vi "Stop FGV_redone.vi"(7 "Mode":enum16{"Set", "Get"}(ring), 8 "Error In":errorcluster, 11 "Set Value":bool) -> (0 "Error Out":errorcluster, 3 "Get Value":bool)   [LabVIEW 2018]
doc: "Functional global variable to stop parallel loops."
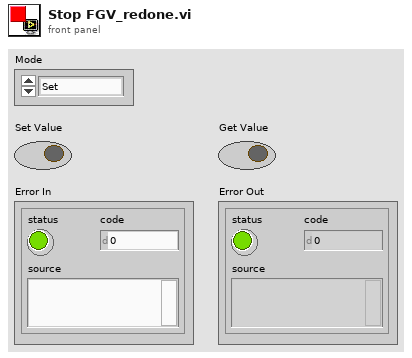
[diagram p1: front panel]
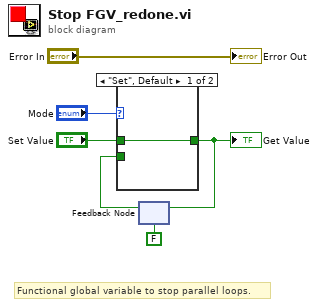
[diagram p0: block diagram]
diagram:
  # "Functional global variable to stop parallel loops."
  n1 = feedback #1(FALSE ("Set Value")) -> (w2:bool)
  n2 = case shown="\"Set\", Default" "Mode" {
    tunnel: "Set Value" -> [w7 _]
    tunnel: [w7 w8] -> w3
    tunnel: w2 -> [_ w8]
    frame "Set", Default {
    }
    frame "Get" {
    }
  }
  "Get Value" <- w3
  n3 = feedback-in #1(w3) -> ()
  "Error Out" <- "Error In"
